vi "create_counter_file.vi"(7 "Data Files Path":path=path "C:/Users/QCC/Documents/Cesium_project/LabVIEW Projects/data/2011_03_02", 8 "error in (no error)":errorcluster, 9 "iteration string":string, 10 "date/time string":string, 11 "Counter in":refnum<class "Counter.lvclass">) -> (0 "error out":errorcluster, 3 "Counter out":refnum<class "Counter.lvclass">)   [LabVIEW 2013, in "Counter.lvclass"]
uses:
  Counter.lvclass
  Counter.lvclass/Counter.ctl
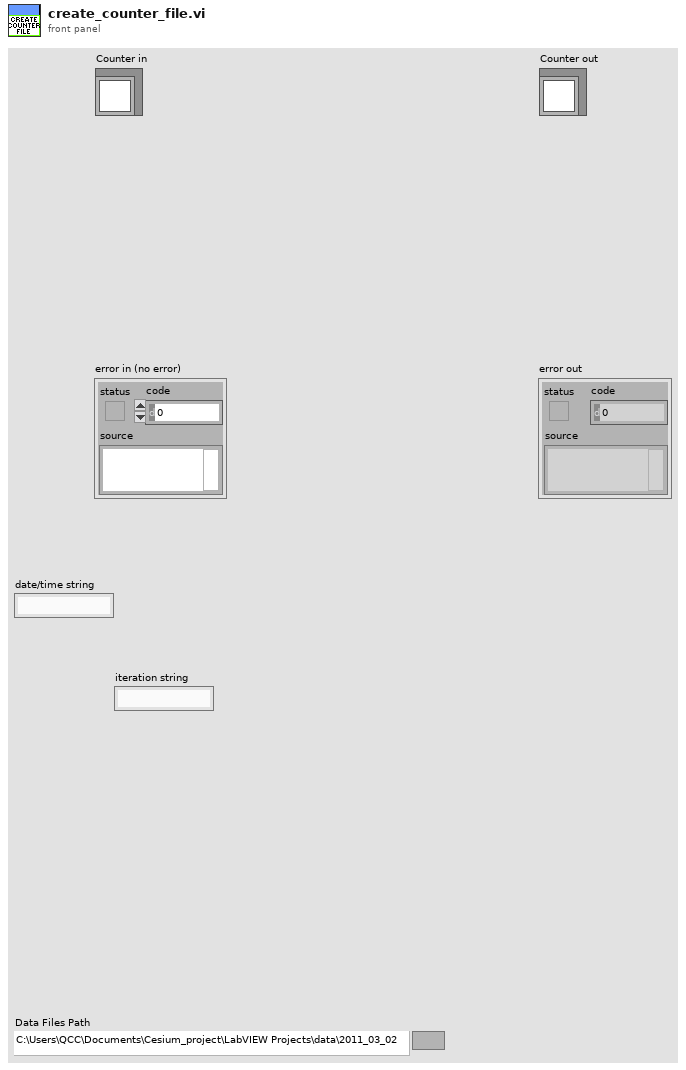
[diagram p1: front panel]
types:
  T1 = cluster{"Counter Channel":tag, "Time-Bin Clock Channel":tag, "Binwidth (ms)":dbl}[]
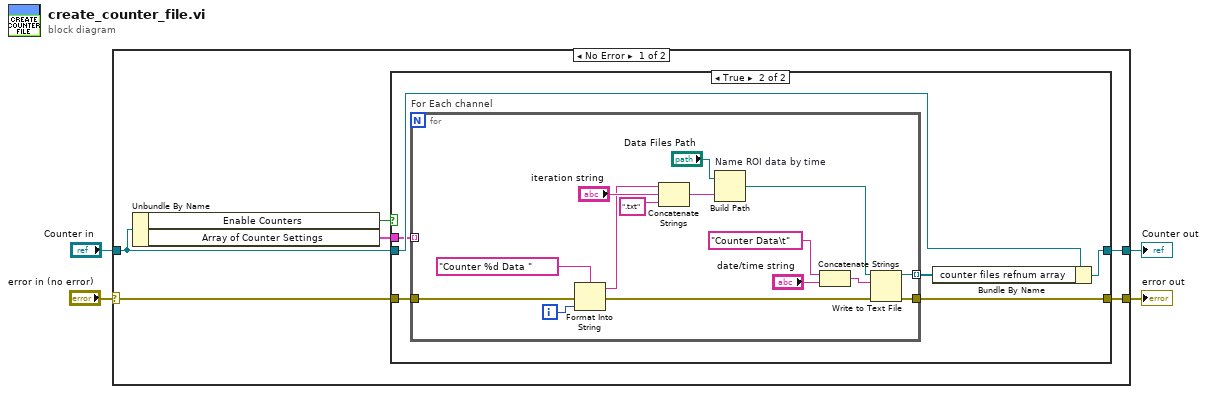
[diagram p0: block diagram]
diagram:
  n1 = case shown="No Error" "error in (no error)" {
    selector: "error in (no error)" -> [w9 w35]
    tunnel: [w10 w35] -> w3
    tunnel: [w6 w34] -> w1
    tunnel: "Counter in" -> [w7 w34]
    frame No Error {
      n2 = Unbundle By Name(w7) -> ("Enable Counters"=w8:bool, "Array of Counter Settings"=w5:T1)
      n3 = case shown="True" w8 {
        tunnel: w9 -> [w12 w18]
        tunnel: [w12 w17] -> w10
        tunnel: w7 -> [w11 w16]
        tunnel: [w11 w15] -> w6
        tunnel: w5 -> [_ w13]
        frame False {
        }
        frame True {
          n4 = for "For Each channel" {
            tunnel: w18 -> [w20]
            tunnel: [w33] -> w17
            tunnel: [w19] -> w14 mode=indexing
            tunnel: w13 -> [_] mode=indexing
            i -> [w32]
            n5 = Format Into String(format string="Counter %d Data ", error in=w20, w32) -> (resulting string=w23:string, error out=w22:errorcluster)  [unwired: 1 in]
            n6 = Concatenate Strings(w23, "iteration string", ".txt" ("string")) -> (w30:string)
            n7 = Build Path "Name ROI data by time"(base path="Data Files Path", name or relative path=w30) -> (appended path=w31:path)
            n8 = Concatenate Strings("Counter Data\t", "date/time string") -> (w26:string)
            n9 = Write to Text File(file (use dialog)=w31, text=w26, error in=w22) -> (refnum out=w19:refnum<file>, error out=w33:errorcluster)  [unwired: 1 in, 1 out]
          }
          n10 = Bundle By Name(cluster=w16, "counter files refnum array"=w14) -> (w15:refnum<class "Counter.lvclass">)
        }
      }
    }
    frame Error {
    }
  }
  "error out" <- w3
  "Counter out" <- w1
